vi "CorrectClimb.vi"(8 "BackEncoder":dbl, 9 "FrontEncoder":dbl, 10 "BackCommand":dbl, 11 "FrontCommand":dbl) -> (2 "BackOutput":dbl, 3 "FrontOutput":dbl)   [LabVIEW 2018]
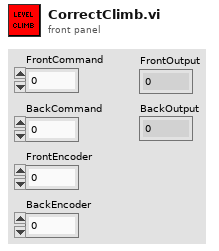
[diagram p1: front panel]
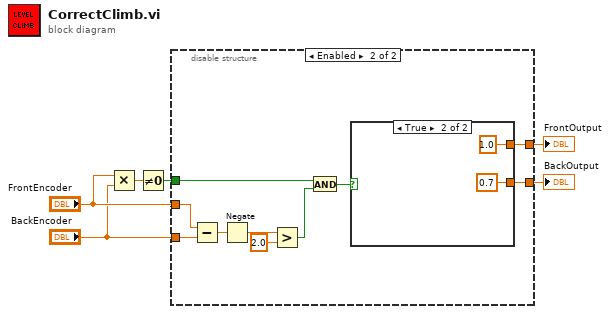
[diagram p0: block diagram]
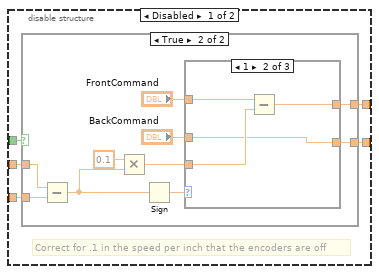
[diagram p2: hidden frame]
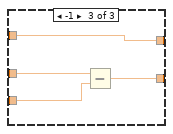
[diagram p5: hidden frame]
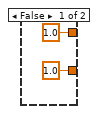
[diagram p6: hidden frame]
diagram:
  n1 = Multiply(x="FrontEncoder", y="BackEncoder") -> (x*y=w5:dbl)
  n2 = Not Equal To 0?(x=w5) -> (x != 0?=w4:bool)
  n3 = disable-structure shown="Enabled" {
    disable-tunnel: "FrontEncoder" -> [w11 w42]
    disable-tunnel: w4 -> [w10 w38]
    disable-tunnel: "BackEncoder" -> [w9 w43]
    disable-tunnel: [w8 w35] -> w2
    disable-tunnel: [w7 w36] -> w1
    frame Disabled {
      # "Correct for .1 in the speed per inch that the encoders are off"
      n4 = case shown="True" w10 {
        tunnel: w9 -> [w12 w23]
        tunnel: w11 -> [w13 w22]
        tunnel: [w12 w15] -> w8
        tunnel: [w13 w14] -> w7
        frame False {
        }
        frame True {
          n5 = Subtract(x=w22, y=w23) -> (x-y=w17:dbl)
          n6 = Multiply(x=0.1, y=w17) -> (x*y=w18:dbl)
          n7 = Sign(1:w17) -> (0:w19:dbl)
          n8 = case shown="1" w19 {
            tunnel: "FrontCommand" -> [w25 w29 w30]
            tunnel: "BackCommand" -> [w24 w26 w33]
            tunnel: [w24 w26 w31] -> w15
            tunnel: [w25 w27 w30] -> w14
            tunnel: w18 -> [_ w28 w32]
            frame 0, Default {
            }
            frame 1 {
              n9 = Subtract(x=w29, y=w28) -> (x-y=w27:dbl)
            }
            frame -1 {
              n10 = Subtract(x=w33, y=w32) -> (x-y=w31:dbl)
            }
          }
        }
      }
    }
    frame Enabled {
      n11 = Subtract(x=w42, y=w43) -> (x-y=w41:dbl)
      n12 = Negate(x=w41) -> (-x=w34:dbl)
      n13 = Greater?(x=w34, y=2.0) -> (0:w39:bool)
      n14 = And(x=w38, y=w39) -> (x .and. y?=w37:bool)
      n15 = case shown="True" w37 {
        tunnel: [1.0 1.0] -> w36
        tunnel: [1.0 0.7] -> w35
        frame False {
        }
        frame True {
        }
      }
    }
  }
  "FrontOutput" <- w1
  "BackOutput" <- w2
